vi "Read Data.vi"(8 "error in":errorcluster, 11 "MC Data in":refnum<class "MC Data.lvclass">) -> (0 "error out":errorcluster, 2 "Data":sgl[](array[numeric]), 3 "MC Data out":refnum<class "MC Data.lvclass">)   [LabVIEW 2019, in "MC Data.lvclass"]
uses:
  MC Data.lvclass
  MC Data.lvclass/MC Data.ctl
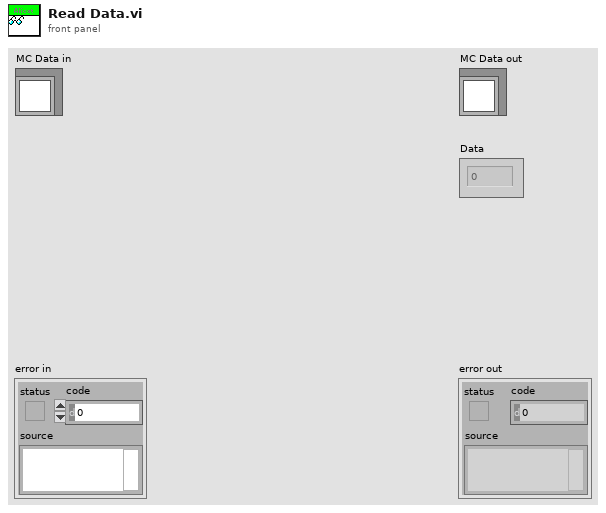
[diagram p1: front panel]
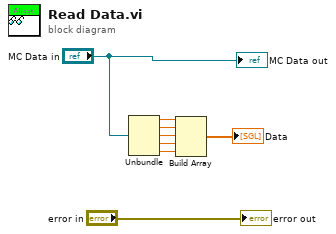
[diagram p0: block diagram]
diagram:
  n1 = Unbundle("MC Data in") -> (w6:sgl, w5:sgl, w4:sgl, w3:sgl, w2:sgl)
  n2 = Build Array(w6, w5, w4, w3, w2) -> (→"Data":sgl[])
  "error out" <- "error in"
  "MC Data out" <- "MC Data in"
